vi "PWM_Lenkung_Array.vi"() -> (0 "8 IR true":bool, 2 "PWM Lenkung":dbl, 3 "Linefollow_Array":bool[](array[boolean]))   [LabVIEW 2016]
doc: "VI berrechnet Abweichung des Linearray zur Mittellinie\n05.04.17_Tloe"
uses:
  <vilib>/myRIO/Instrument Drivers/Onboard IO/DIO/typedefs/DIO Reference.ctl
  <vilib>/myRIO/Common/Instrument Driver Framework/Utilities/typedefs/myRIO Generic Hardware Reference.ctl
  <vilib>/myRIO/Common/Instrument Driver Framework/Utilities/typedefs/Hardware Version Enum.ctl
  <vilib>/myRIO/Common/Instrument Driver Framework/Utilities/typedefs/myRIO v1.0 Reference.ctl
  <vilib>/myRIO/Common/Instrument Driver Framework/Utilities/typedefs/Generic FPGA Reference.ctl
  <vilib>/myRIO/Common/Instrument Driver Framework/myRIO v1.0/DIO/typedefs/DIO Channels List.ctl
  <vilib>/myRIO/Common/Instrument Driver Framework/myRIO v1.0/DIO/typedefs/DIO Channels Enum.ctl
  <vilib>/userdefined/High Color/nirio_resource_hc.ctl
  <vilib>/myRIO/Common/Instrument Driver Framework/Utilities/vis/Is FPGA Ref Available.vi
  <vilib>/myRIO/Common/Instrument Driver Framework/myRIO v1.0/DIO/vis/myRIO v1.1 Open DIO.vi
  <vilib>/myRIO/Instrument Drivers/Onboard IO/DIO/vis/Read.vi
  <vilib>/myRIO/Common/Instrument Driver Framework/Utilities/vis/Validate Channels.vi
  <vilib>/myRIO/Common/Instrument Driver Framework/myRIO v1.0/DIO/vis/myRIO v1.0 Reserve DIO.vi
  <vilib>/myRIO/Common/Instrument Driver Framework/myRIO v1.0/Resource Manager/vis/myRIO v1.0 Reserve Channel List.vi
  <vilib>/myRIO/Common/Instrument Driver Framework/myRIO v1.0/DIO/vis/myRIO v1.0 Build MUX Configuration DIO.vi
  <vilib>/myRIO/Common/Instrument Driver Framework/myRIO v1.0/Resource Manager/vis/myRIO v1.0 Reserve Channel.vi
  <vilib>/myRIO/Common/Instrument Driver Framework/myRIO v1.0/Resource Manager/vis/myRIO v1.0 Unreserve Channel.vi
  <vilib>/myRIO/Common/Instrument Driver Framework/myRIO v1.0/Resource Manager/vis/myRIO v1.0 Create Configuration List.vi
  <vilib>/myRIO/Common/Instrument Driver Framework/myRIO v1.0/Resource Manager/vis/myRIO v1.0 Build Mutex Name.vi
  <vilib>/Utility/VariantDataType/GetNumericInfo.vi
  <vilib>/Utility/error.llb/Error Cluster From Error Code.vi
  <vilib>/myRIO/Common/Instrument Driver Framework/myRIO v1.0/myRIO v1.1 Open.vi
  <vilib>/myRIO/Common/Instrument Driver Framework/Utilities/vis/IO Manager.vi
  <vilib>/myRIO/Common/Instrument Driver Framework/Utilities/vis/Configuration Manager.vi
  <vilib>/myRIO/Common/Instrument Driver Framework/myRIO v1.0/Resource Manager/vis/myRIO v1.0 Configure IO.vi
  <vilib>/myRIO/Common/Instrument Driver Framework/myRIO v1.0/myRIO v1.0 Close.vi
  <vilib>/myRIO/Common/Instrument Driver Framework/myRIO v1.0/DIO/vis/myRIO v1.0 Read DIO.vi
  <vilib>/addons/control/pid/pid.llb/PID (DBL).vi
  <vilib>/myRIO/Express VI/Onboard IO/DI/DI Express VI.xnode
  <vilib>/myRIO/Instrument Drivers/Onboard IO/DIO/vis/myRIO DIO Open.xnode
  <vilib>/myRIO/Instrument Drivers/Onboard IO/DIO/DIO.lvlib
  <vilib>/addons/control/pid/NI_PID_pid.lvlib
panel:
  in  "PID gains":T1={"proportional gain (Kc)"=0.61, "integral time (Ti, min)"=0.08, "derivative time (Td, min)"=0.32}
  in  "Sensorarray\nZusatzwerte":dbl[](array[numeric])=[4.0, 3.0, 2.0, 1.0, -1.0, -2.0, -3.0, -4.0]
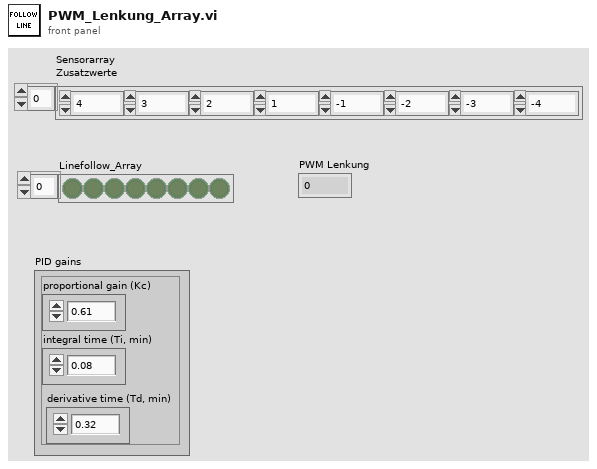
[diagram p1: front panel]
types:
  T1 = cluster{"proportional gain (Kc)":dbl, "integral time (Ti, min)":dbl, "derivative time (Td, min)":dbl}
  T2 = cluster{"A/DIO0 (Pin 11)":bool, "A/DIO1 (Pin 13)":bool, "A/DIO2 (Pin 15)":bool, "A/DIO3 (Pin 17)":bool, "A/DIO4 (Pin 19)":bool, "A/DIO5 (Pin 21)":bool, "A/DIO6 (Pin 23)":bool, "A/DIO7 (Pin 25)":bool}
  T3 = cluster{"A/DIO0 (Pin 11)":i16, "A/DIO1 (Pin 13)":i16, "A/DIO2 (Pin 15)":i16, "A/DIO3 (Pin 17)":i16, "A/DIO4 (Pin 19)":i16, "A/DIO5 (Pin 21)":i16, "A/DIO6 (Pin 23)":i16, "A/DIO7 (Pin 25)":i16}
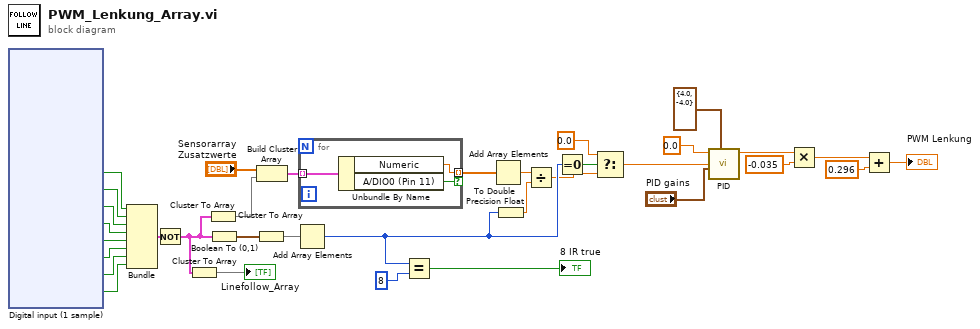
[diagram p0: block diagram]
diagram:
  n1 = xnode "Digital input (1 sample)"() -> ("A/DIO0 (Pin 11)"=w20:bool, "A/DIO1 (Pin 13)"=w21:bool, "A/DIO2 (Pin 15)"=w22:bool, "A/DIO3 (Pin 17)"=w23:bool, "A/DIO4 (Pin 19)"=w24:bool, "A/DIO5 (Pin 21)"=w25:bool, "A/DIO6 (Pin 23)"=w26:bool, "A/DIO7 (Pin 25)"=w27:bool)  [unwired: 1 in, 1 out]
  n2 = Bundle("A/DIO0 (Pin 11)"=w20, "A/DIO1 (Pin 13)"=w21, "A/DIO2 (Pin 15)"=w22, "A/DIO3 (Pin 17)"=w23, "A/DIO4 (Pin 19)"=w24, "A/DIO5 (Pin 21)"=w25, "A/DIO6 (Pin 23)"=w26, "A/DIO7 (Pin 25)"=w27) -> (w15:T2)  [unwired: 1 in]
  n3 = Not(x=w15) -> (.not. x?=w33:T2)
  n4 = Cluster To Array(cluster=w33) -> (array=→"Linefollow_Array":bool[])
  n5 = Cluster To Array(cluster=w33) -> (array=w16:bool[])
  n6 = Boolean To (0,1)(Boolean=w33) -> (0, 1=w29:T3)
  n7 = Cluster To Array(cluster=w29) -> (array=w30:i16[])
  n8 = Build Cluster Array("Sensorarray\nZusatzwerte", w16) -> (w17:cluster{"Numeric":dbl, "A/DIO0 (Pin 11)":bool}[])
  n9 = Add Array Elements(numeric array=w30) -> (sum=w32:i16)
  n10 = for {
    tunnel: w17 -> [w37] mode=indexing
    tunnel: [w36] -> w19 mode=indexing if=w35
    n11 = Unbundle By Name(w37) -> ("Numeric"=w36:dbl, "A/DIO0 (Pin 11)"=w35:bool)
  }
  n12 = Equal?(x=w32, y=i16 8) -> (x = y?=→"8 IR true":bool)
  n13 = Add Array Elements(numeric array=w19) -> (sum=w28:dbl)
  n14 = To Double Precision Float(number=w32) -> (double precision float=w34:dbl)
  n15 = Divide(x=w28, y=w34) -> (x/y=w13:dbl)
  n16 = Equal To 0?(x=w32) -> (x = 0?=w11:bool)
  n17 = Select(t=0.0, s=w11, f=w13) -> (s? t:f=w3:dbl)
  n18 = call-poly <vilib>:"PID.vi"("output range"=cluster{"output high":dbl, "output low":dbl} {"output high"=4.0, "output low"=-4.0}, "PID gains"="PID gains", "process variable"=w3, "setpoint"=0.0) -> ("output"=w8:dbl)  [unwired: 6 in, 1 out]
  n19 = Multiply(x=w8, y=-0.035) -> (x*y=w9:dbl)
  n20 = Add(x=w9, y=0.296) -> (x+y=→"PWM Lenkung":dbl)
